vi "HXG2pidFGV.vi"(0 "Liq PID Resets":T1, 1 "AF PID Resets":T2, 2 "PIDfgvCtrl":T7, 5 "PIDon-off In":T6, 7 "PID Gains Array":T4, 9 "PID Ref cluster":T5, 11 "error in (no error)":errorcluster, 12 "PID Ctrls":T3) -> (3 "Air PID Resets":T2, 4 "Liq PID Resets":T1, 6 "PIDon-off":T6, 8 "PID Gains Array Out":T4, 10 "PID Refs Out":T5, 14 "PID Ctrls Out":T3, 15 "error out":errorcluster)   [LabVIEW 2012]
uses:
  HXG2pid.ctl
  Controls/HXG2_PIDon-off.ctl
  CondensingVIs/PIDCtrl/HXG2_References.ctl
  Controls/HXG2_PIDgains_Array.ctl
  Controls/HXG2_PIDctrlsOUT.ctl
  Controls/HXG2_AirPIDresets.ctl
  Controls/HXG2_LiqPIDresets.ctl
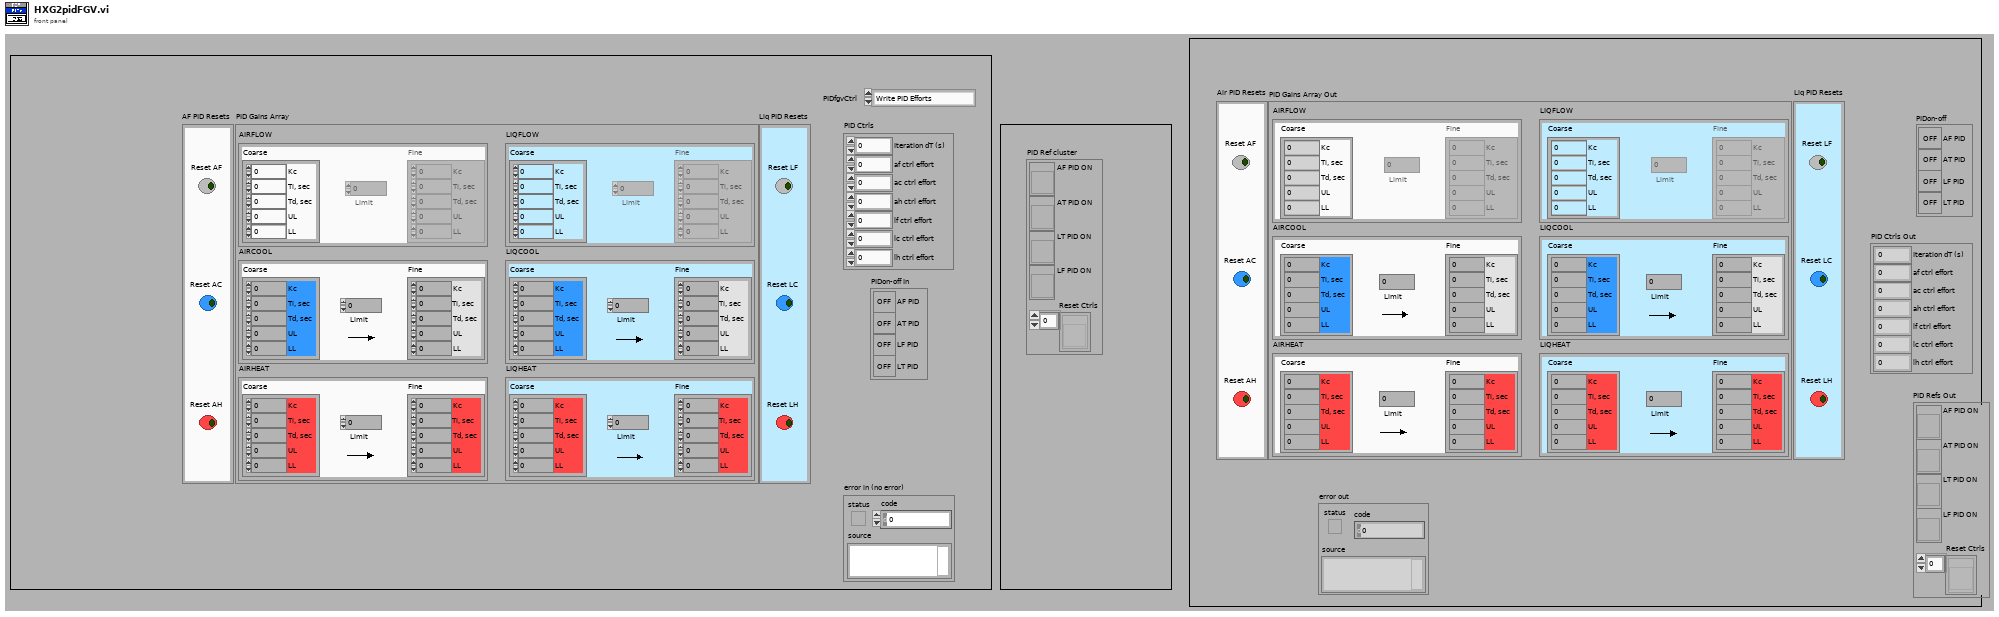
[diagram p1: front panel]
types:
  T1 = typedef "HXG2_LiqPIDresets.ctl" = cluster{"Reset LF":bool, "Reset LC":bool, "Reset LH":bool}
  T2 = typedef "HXG2_AirPIDresets.ctl" = cluster{"Reset AF":bool, "Reset AC":bool, "Reset AH":bool}
  T3 = typedef "HXG2_PIDctrlsOUT.ctl" = cluster{"Iteration dT (s)":dbl, "af ctrl effort":dbl, "ac ctrl effort":dbl, "ah ctrl effort":dbl, "lf ctrl effort":dbl, "lc ctrl effort":dbl, "lh ctrl effort":dbl}
  T4 = typedef "HXG2_PIDgains_Array.ctl" = cluster{"AIRFLOW":cluster{"Coarse":cluster{"Kc":dbl, "Ti, sec":dbl, "Td, sec":dbl, "UL":dbl, "LL":dbl}, "Fine":cluster{"Kc":dbl, "Ti, sec":dbl, "Td, sec":dbl, "UL":dbl, "LL":dbl}, "Limit":dbl}, "AIRCOOL":cluster{"Coarse":cluster{"Kc":dbl, "Ti, sec":dbl, "Td, sec":dbl, "UL":dbl, "LL":dbl}, "Fine":cluster{"Kc":dbl, "Ti, sec":dbl, "Td, sec":dbl, "UL":dbl, "LL":dbl}, "Limit":dbl}, "AIRHEAT":cluster{"Coarse":cluster{"Kc":dbl, "Ti, sec":dbl, "Td, sec":dbl, "UL":dbl, "LL":dbl}, "Fine":cluster{"Kc":dbl, "Ti, sec":dbl, "Td, sec":dbl, "UL":dbl, "LL":dbl}, "Limit":dbl}, "LIQFLOW":cluster{"Coarse":cluster{"Kc":dbl, "Ti, sec":dbl, "Td, sec":dbl, "UL":dbl, "LL":dbl}, "Fine":cluster{"Kc":dbl, "Ti, sec":dbl, "Td, sec":dbl, "UL":dbl, "LL":dbl}, "Limit":dbl}, "LIQCOOL":cluster{"Coarse":cluster{"Kc":dbl, "Ti, sec":dbl, "Td, sec":dbl, "UL":dbl, "LL":dbl}, "Fine":cluster{"Kc":dbl, "Ti, sec":dbl, "Td, sec":dbl, "UL":dbl, "LL":dbl}, "Limit":dbl}, "LIQHEAT":cluster{"Coarse":cluster{"Kc":dbl, "Ti, sec":dbl, "Td, sec":dbl, "UL":dbl, "LL":dbl}, "Fine":cluster{"Kc":dbl, "Ti, sec":dbl, "Td, sec":dbl, "UL":dbl, "LL":dbl}, "Limit":dbl}}
  T5 = typedef "HXG2_References.ctl" = cluster{"AF PID ON":refnum<vi>, "AT PID ON":refnum<vi>, "LT PID ON":refnum<vi>, "LF PID ON":refnum<vi>, "Reset Ctrls":refnum<vi>[]}
  T6 = typedef "HXG2_PIDon-off.ctl" = cluster{"AF PID":bool, "AT PID":bool, "LF PID":bool, "LT PID":bool}
  T7 = typedef "HXG2pid.ctl" = enum16{"Write PID Efforts", "Write PID On-Off", "Pass", "Write PID Refs", "Write PID pop-up", "Wrt PID Resets"}
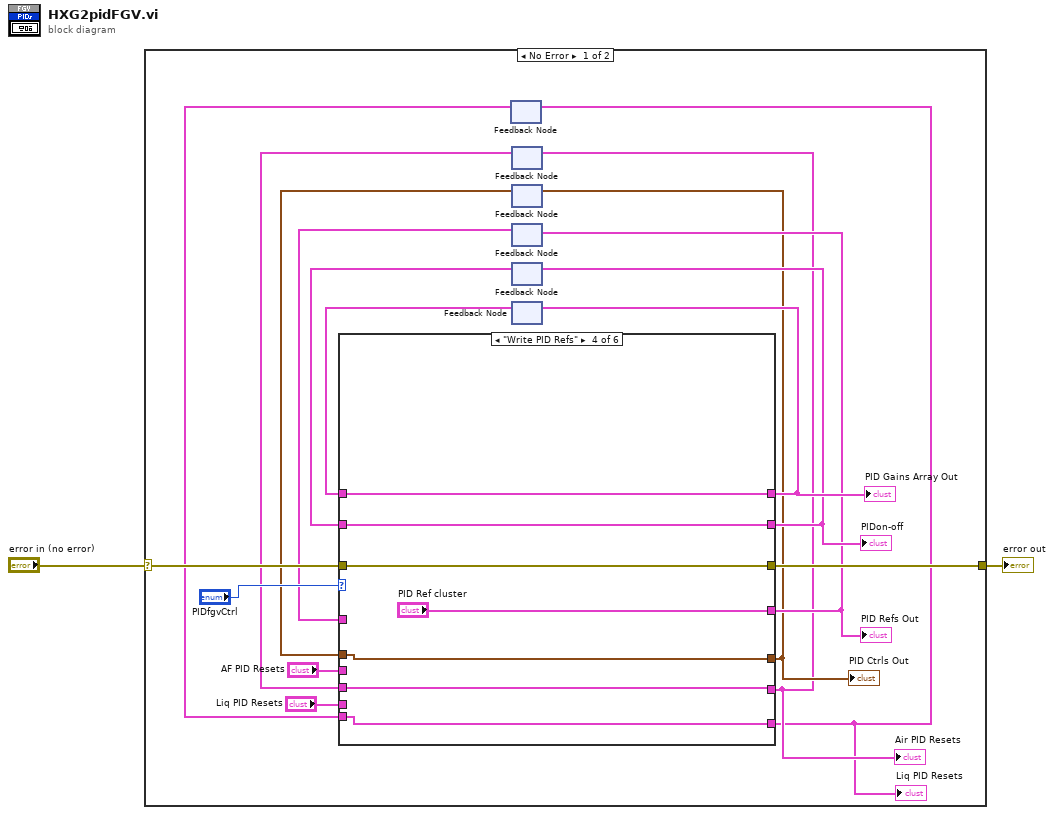
[diagram p0: block diagram]
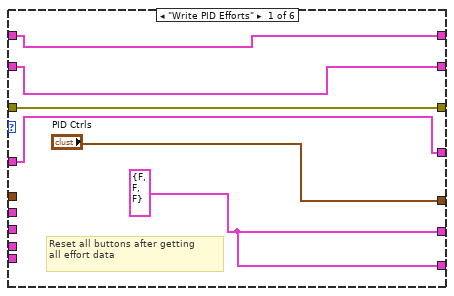
[diagram p2: hidden frame]
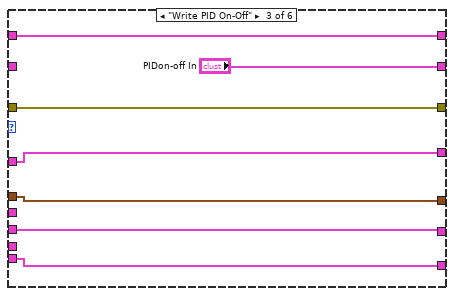
[diagram p4: hidden frame]
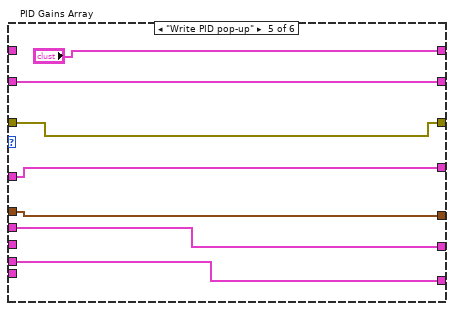
[diagram p5: hidden frame]
diagram:
  n1 = case shown="No Error" "error in (no error)" {
    selector: "error in (no error)" -> [w19 w61]
    tunnel: [w18 w61] -> w1
    frame No Error {
      n2 = feedback #1() -> (w7:T1)  [unwired: 1 in]
      n3 = feedback #2() -> (w8:T2)  [unwired: 1 in]
      n4 = feedback #3() -> (w10:T3)  [unwired: 1 in]
      n5 = feedback #4() -> (w11:T5)  [unwired: 1 in]
      n6 = feedback #5() -> (w15:T6)  [unwired: 1 in]
      n7 = feedback #6() -> (w17:T4)  [unwired: 1 in]
      n8 = case shown="\"Write PID Refs\"" "PIDfgvCtrl" {
        tunnel: w19 -> [w25 w31 w37 w42 w50 w57]
        tunnel: [w25 w31 w37 w42 w50 w57] -> w18
        tunnel: [w22 w32 w38 w46 "PID Gains Array" w56] -> w14
        tunnel: w17 -> [w22 w32 w38 w46 _ w56]
        tunnel: [w24 w30 "PIDon-off In" w45 w53 w60] -> w13
        tunnel: w15 -> [w24 w30 _ w45 w53 w60]
        tunnel: [w23 w29 w35 "PID Ref cluster" w52 w59] -> w12
        tunnel: w11 -> [w23 w29 w35 _ w52 w59]
        tunnel: ["PID Ctrls" w28 w36 w44 w51 w58] -> w9
        tunnel: w10 -> [_ w28 w36 w44 w51 w58]
        tunnel: [w20 w27 w34 w41 w48 w55] -> w4
        tunnel: w8 -> [_ w27 w34 w41 _ _]
        tunnel: [w20 w26 w33 w40 w47 w54] -> w3
        tunnel: w7 -> [_ w26 w33 w40 _ w54]
        tunnel: "AF PID Resets" -> [_ _ _ _ w48 w55]
        tunnel: "Liq PID Resets" -> [_ _ _ _ w47 _]
        frame "Write PID Efforts" {
          w20 = T2 {"Reset AF"=FALSE, "Reset AC"=FALSE, "Reset AH"=FALSE} ("AF PID Resets")
          # "Reset all buttons after getting\nall effort data"
        }
        frame "Pass" {
        }
        frame "Write PID On-Off" {
        }
        frame "Write PID Refs" {
        }
        frame "Write PID pop-up" {
        }
        frame "Wrt PID Resets" {
          # "So that we can write Upper limits in positive values in the UI\nthe switch to negative numbers is made here"
        }
      }
      "PIDon-off" <- w13
      "PID Refs Out" <- w12
      "PID Gains Array Out" <- w14
      "PID Ctrls Out" <- w9
      "Air PID Resets" <- w4
      "Liq PID Resets" <- w3
      n9 = feedback-in #1(w3) -> ()
      n10 = feedback-in #2(w4) -> ()
      n11 = feedback-in #3(w9) -> ()
      n12 = feedback-in #4(w12) -> ()
      n13 = feedback-in #5(w13) -> ()
      n14 = feedback-in #6(w14) -> ()
    }
    frame Error {
    }
  }
  "error out" <- w1
